vi "Read Destiny.vi"(8 "error in (no error)":errorcluster, 11 "GoToSkill in":refnum<class "GoToSkill.lvclass">) -> (0 "error out":errorcluster, 2 "Destiny":dbl[](array[numeric]), 3 "GoToSkill out":refnum<class "GoToSkill.lvclass">)   [LabVIEW 2023, in "GoToSkill.lvclass"]
uses:
  GoToSkill.lvclass
  GoToSkill.lvclass/GoToSkill.ctl
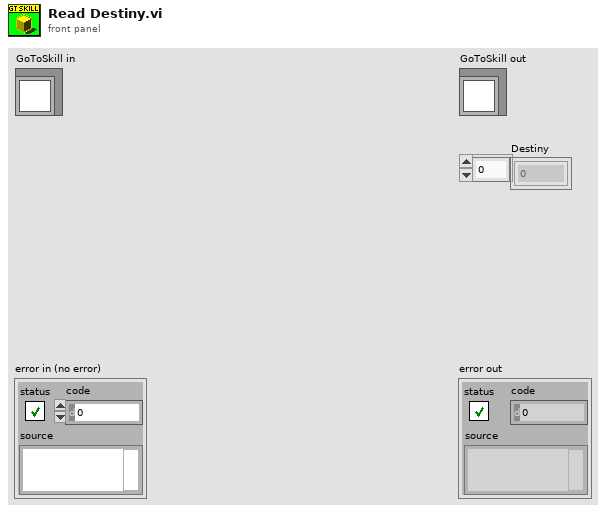
[diagram p1: front panel]
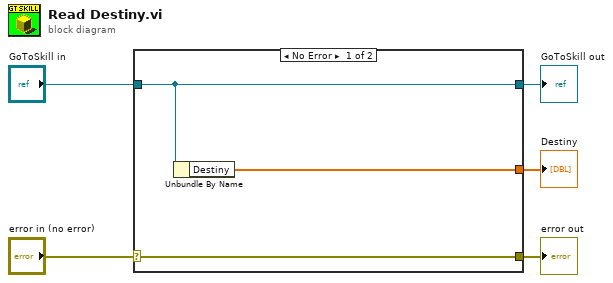
[diagram p0: block diagram]
diagram:
  n1 = case shown="No Error" "error in (no error)" {
    selector: "error in (no error)" -> [w8 w9]
    tunnel: [w8 w9] -> w4
    tunnel: [w7 w10] -> w2
    tunnel: "GoToSkill in" -> [w7 w10]
    tunnel: [w6 _] -> w1
    frame No Error {
      n2 = Unbundle By Name(w7) -> ("Destiny"=w6:dbl[])
    }
    frame Error {
    }
  }
  "error out" <- w4
  "GoToSkill out" <- w2
  "Destiny" <- w1
